vi "hl_magstim_set_intensity_A.vi"(2 "Pause":i32=50, 3 "Power In":i32) -> (0 "dup VISA\nresource\nname":refnum<visa-resource-name>, 1 "Power Out":i32)   [LabVIEW 2014]
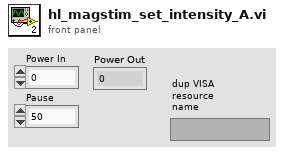
[diagram p1: front panel]
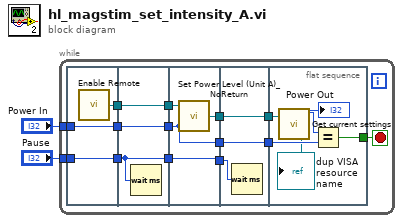
[diagram p0: block diagram]
diagram:
  n1 = while {
    tunnel: "Power In" -> [w14]
    tunnel: "Pause" -> [w6]
    stop <- w7 stop-if-true
    n2 = flat-sequence {
      tunnel: [w19] -> w16
      tunnel: w14 -> [w18]
      tunnel: [w18] -> w13
      tunnel: w6 -> [w17]
      tunnel: [w17] -> w5
      tunnel: w16 -> [w22]
      tunnel: [w22] -> w15
      tunnel: w13 -> [w21]
      tunnel: [w21] -> w12
      tunnel: w5 -> [w20]
      tunnel: [w20] -> w3
      tunnel: w15 -> [w26]
      tunnel: [w25] -> w11
      tunnel: w12 -> [w24]
      tunnel: [w24] -> w9
      tunnel: [w23] -> w4
      tunnel: w3 -> [w23]
      tunnel: w11 -> [w29]
      tunnel: [w29] -> w10
      tunnel: w9 -> [w28]
      tunnel: [w28] -> w8
      tunnel: w4 -> [w27]
      tunnel: w10 -> [w34]
      tunnel: w8 -> [w32]
      tunnel: [w31] -> w7
      frame #0 {
        n3 = call "Enable Remote.vi"() -> ("dup VISA resource name"=w19:refnum<visa-resource-name>)  [unwired: 1 in]
      }
      frame #1 {
        n4 = Wait (ms)(milliseconds to wait=w20) -> ()  [unwired: 1 out]
      }
      frame #2 {
        n5 = call "Set Power Level (Unit A)_NoReturn.vi"("Power Level (% of threshold)"=w24, "VISA resource name"=w26) -> ("dup VISA resource name"=w25:refnum<visa-resource-name>)  [unwired: 1 in]
      }
      frame #3 {
        n6 = Wait (ms)(milliseconds to wait=w27) -> ()  [unwired: 1 out]
      }
      frame #4 {
        n7 = call "Get current settings.vi"("VISA resource name"=w34) -> ("dup VISA resource name"=→"dup VISA\nresource\nname":refnum<visa-resource-name>, "Power Unit A"=w33:i32)  [unwired: 4 out]
        "Power Out" <- w33
        n8 = Equal?(x=w33, y=w32) -> (x = y?=w31:bool)
      }
    }
  }
